vi "get_commands.vi"(8 "error in (no error)":errorcluster, 11 "Protocol_Generic in":refnum<class "Protocol_Generic.lvclass">) -> (0 "error out":errorcluster, 2 "commands":refnum<class "command_generic.lvclass">[](array[class]), 3 "Protocol_Generic out":refnum<class "Protocol_Generic.lvclass">)   [LabVIEW 2015, in "Protocol_Generic.lvclass"]
uses:
  Protocol_Generic.lvclass
  command/command_generic.lvclass
  Protocol_Generic.lvclass/Protocol_Generic.ctl
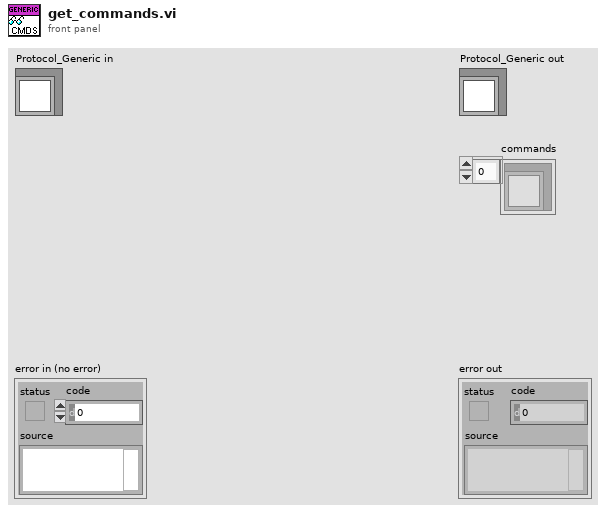
[diagram p1: front panel]
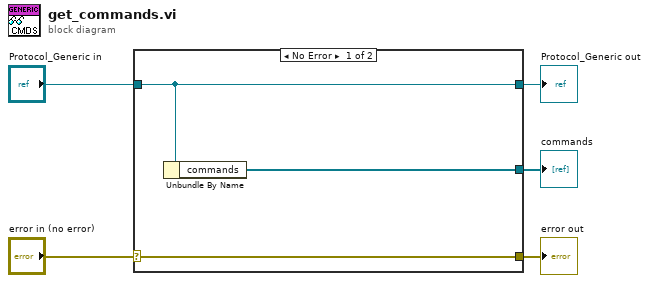
[diagram p0: block diagram]
diagram:
  n1 = case shown="No Error" "error in (no error)" {
    selector: "error in (no error)" -> [w8 w9]
    tunnel: [w8 w9] -> w4
    tunnel: [w7 w10] -> w2
    tunnel: "Protocol_Generic in" -> [w7 w10]
    tunnel: [w6 _] -> w1
    frame No Error {
      n2 = Unbundle By Name(w7) -> ("commands"=w6:refnum<class "command_generic.lvclass">[])
    }
    frame Error {
    }
  }
  "error out" <- w4
  "Protocol_Generic out" <- w2
  "commands" <- w1
